vi "VI Tree.vi"   [LabVIEW 2012, in "Phidget RFID.lvlib"]
doc: "${RFID:VITreeHeader}"
uses:
  <instrlib>/Phidgets/Phidget RFID/Phidget RFID.lvlib
  <instrlib>/Phidgets/Phidget RFID/Public/RFIDStart.vi
  <instrlib>/Phidgets/Phidget RFID/Public/RFIDOpen.vi
  <instrlib>/Phidgets/Phidget RFID/Public/RFIDClose.vi
panel:
  # "(c) 2015 Phidgets Inc..  ALL RIGHTS RESERVED."
  # "SEE DIAGRAM\nFOR VI TREE."
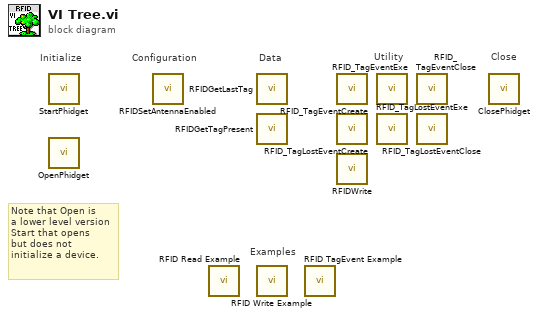
[diagram p0: block diagram]
diagram:
  # "Note that Open is\na lower level version\nStart that opens\nbut does not \ninitialize a device."
  # "Examples"
  # "Configuration"
  # "Utility"
  # "Data"
  # "Close"
  # "Initialize"
  n1 = call-poly <instrlib>:"StartPhidget.vi"() -> ()  [unwired: 12 in, 4 out]
  n2 = call-poly <instrlib>:"OpenPhidget.vi"() -> ()  [unwired: 8 in, 4 out]
  n3 = call <instrlib>:"RFIDSetAntennaEnabled.vi"() -> ()  [unwired: 9 in, 2 out]
  n4 = call <instrlib>:"RFID Read Example.vi"() -> ()  [unwired: 12 in]
  n5 = call <instrlib>:"RFIDGetLastTag.vi"() -> ()  [unwired: 8 in, 4 out]
  n6 = call <instrlib>:"RFIDGetTagPresent.vi"() -> ()  [unwired: 8 in, 3 out]
  n7 = call <instrlib>:"RFID Write Example.vi"() -> ()  [unwired: 12 in]
  n8 = call <instrlib>:"RFID TagEvent Example.vi"() -> ()  [unwired: 12 in]
  n9 = call <instrlib>:"RFID_TagEventCreate.vi"() -> ()  [unwired: 9 in, 3 out]
  n10 = call <instrlib>:"RFID_TagLostEventCreate.vi"() -> ()  [unwired: 9 in, 3 out]
  n11 = call <instrlib>:"RFIDWrite.vi"() -> ()  [unwired: 14 in, 2 out]
  n12 = call <instrlib>:"RFID_TagEventExe.vi"() -> ()  [unwired: 8 in, 8 out]
  n13 = call <instrlib>:"RFID_TagLostEventExe.vi"() -> ()  [unwired: 8 in, 8 out]
  n14 = call <instrlib>:"RFID_TagEventClose.vi"() -> ()  [unwired: 10 in, 2 out]
  n15 = call <instrlib>:"RFID_TagLostEventClose.vi"() -> ()  [unwired: 10 in, 2 out]
  n16 = call-poly <instrlib>:"ClosePhidget.vi"() -> ()  [unwired: 11 in, 1 out]
